vi "Slave_P.vi"() -> ()   [LabVIEW 2017, in "Konfiguracja.lvlib"]
uses:
  Libraries/Konfiguracja/Konfiguracja.lvlib
  Controls/Enum_SM_read_input_write.ctl
  <vilib>/Utility/config.llb/NI_LVConfig.lvlib
panel:
  in  "System Tab":enum32{"Termometry i paliwo"}(tab)
  in  "Etykiety P1-6":T1
  in  "Ratio 6":dbl min=0.0 step=1.0
  in  "Ratio 5":dbl min=0.0 step=1.0
  in  "Ratio 4":dbl min=0.0 step=1.0
  in  "Ratio 3":dbl min=0.0 step=1.0
  in  "Ratio 2":dbl min=0.0 step=1.0
  in  "Ratio 1":dbl min=0.0 step=1.0
  in  "Stan 6":dbl min=0.0 step=1.0
  in  "Stan 5":dbl min=0.0 step=1.0
  in  "Stan 4":dbl min=0.0 step=1.0
  in  "Stan 3":dbl min=0.0 step=1.0
  in  "Stan 2":dbl min=0.0 step=1.0
  in  "Stan 1":dbl min=0.0 step=1.0
  in  "Paliwo 6":bool
  in  "Paliwo 5":bool
  in  "Paliwo 4":bool
  in  "Paliwo 3":bool
  in  "Paliwo 2":bool
  in  "Paliwo 1":bool caption="Termometr 1"
  in  "Moduł aktywny":bool
  in  "Identyfikator slave'a":dbl=2.0 min=2.0 max=127.0 step=1.0
  in  "Copy":bool
  in  "Save":bool
  # "Etykieta"
  # "Stan licznika"
  # "Ratio"
  # "Kopiuje wartośc zadaną z \npola 1 do pozostałych"
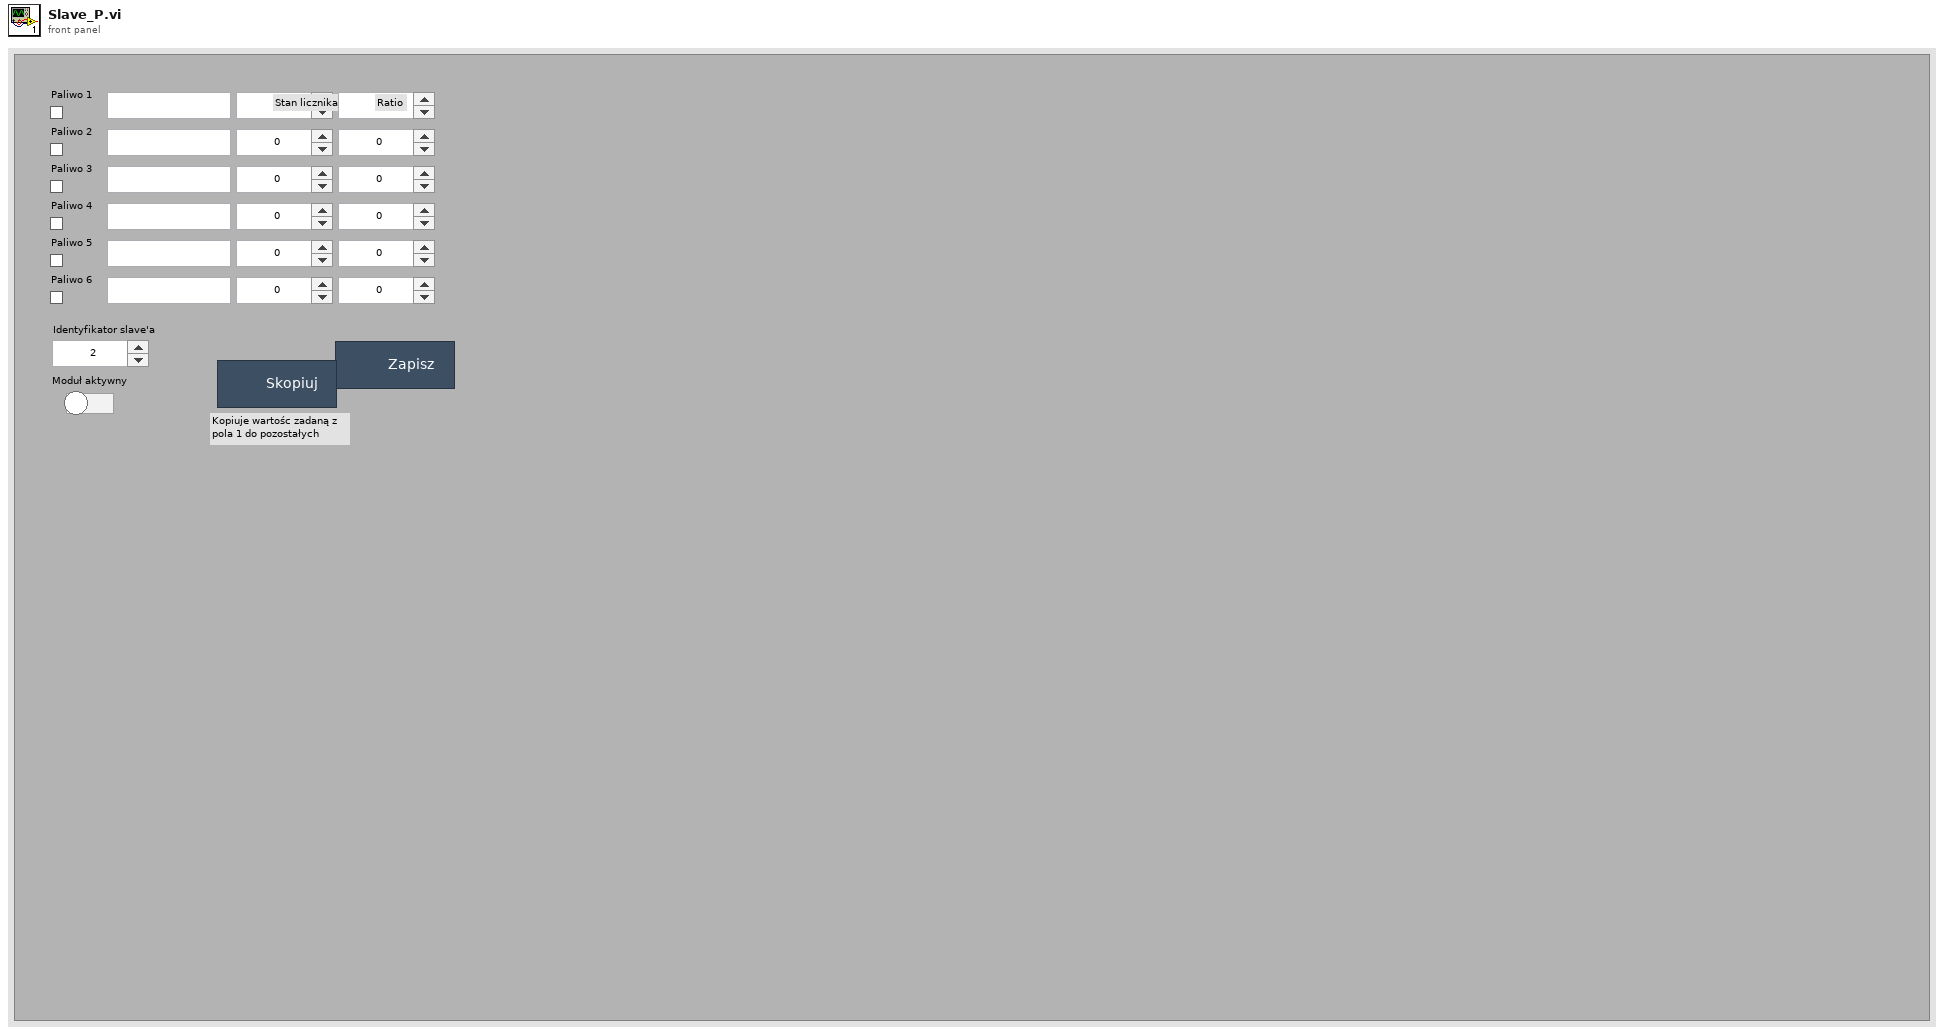
[diagram p1: front panel]
types:
  T1 = cluster{"Paliwo 1":string, "Paliwo 2":string, "Paliwo 3":string, "Paliwo 4":string, "Paliwo 5":string, "Paliwo 6":string}
  T2 = typedef "Konfiguracja.lvlib/Enum_SM_read_input_write.ctl" = enum16{"Load", "Wait for input", "Input", "Copy", "Write", "Exit"}
  T3 = cluster{bool, "P_Sx":cluster{"Stan 1":dbl, "Stan 2":dbl, "Stan 3":dbl, "Stan 4":dbl, "Stan 5":dbl, "Stan 6":dbl}, "P_Rx":cluster{"Ratio 1":dbl, "Ratio 2":dbl, "Ratio 3":dbl, "Ratio 4":dbl, "Ratio 5":dbl, "Ratio 6":dbl}, "Px":cluster{"Paliwo 1":bool, "Paliwo 2":bool, "Paliwo 3":bool, "Paliwo 4":bool, "Paliwo 5":bool, "Paliwo 6":bool}}
  T4 = cluster{"Stan 1":dbl, "Stan 2":dbl, "Stan 3":dbl, "Stan 4":dbl, "Stan 5":dbl, "Stan 6":dbl}
  T5 = cluster{"Ratio 1":dbl, "Ratio 2":dbl, "Ratio 3":dbl, "Ratio 4":dbl, "Ratio 5":dbl, "Ratio 6":dbl}
  T6 = cluster{"Paliwo 1":bool, "Paliwo 2":bool, "Paliwo 3":bool, "Paliwo 4":bool, "Paliwo 5":bool, "Paliwo 6":bool}
  T7 = cluster{cluster{"Paliwo 1":bool, "Paliwo 2":bool, "Paliwo 3":bool, "Paliwo 4":bool, "Paliwo 5":bool, "Paliwo 6":bool}, cluster{"Ratio 1":dbl, "Ratio 2":dbl, "Ratio 3":dbl, "Ratio 4":dbl, "Ratio 5":dbl, "Ratio 6":dbl}, cluster{"Stan 1":dbl, "Stan 2":dbl, "Stan 3":dbl, "Stan 4":dbl, "Stan 5":dbl, "Stan 6":dbl}, "Moduł aktywny":bool, "Etykiety P1-6":cluster{"Paliwo 1":string, "Paliwo 2":string, "Paliwo 3":string, "Paliwo 4":string, "Paliwo 5":string, "Paliwo 6":string}}
  T8 = typedef "NI_LVConfig.lvlib/Config Data RefNum.ctl" = refnum<k1>
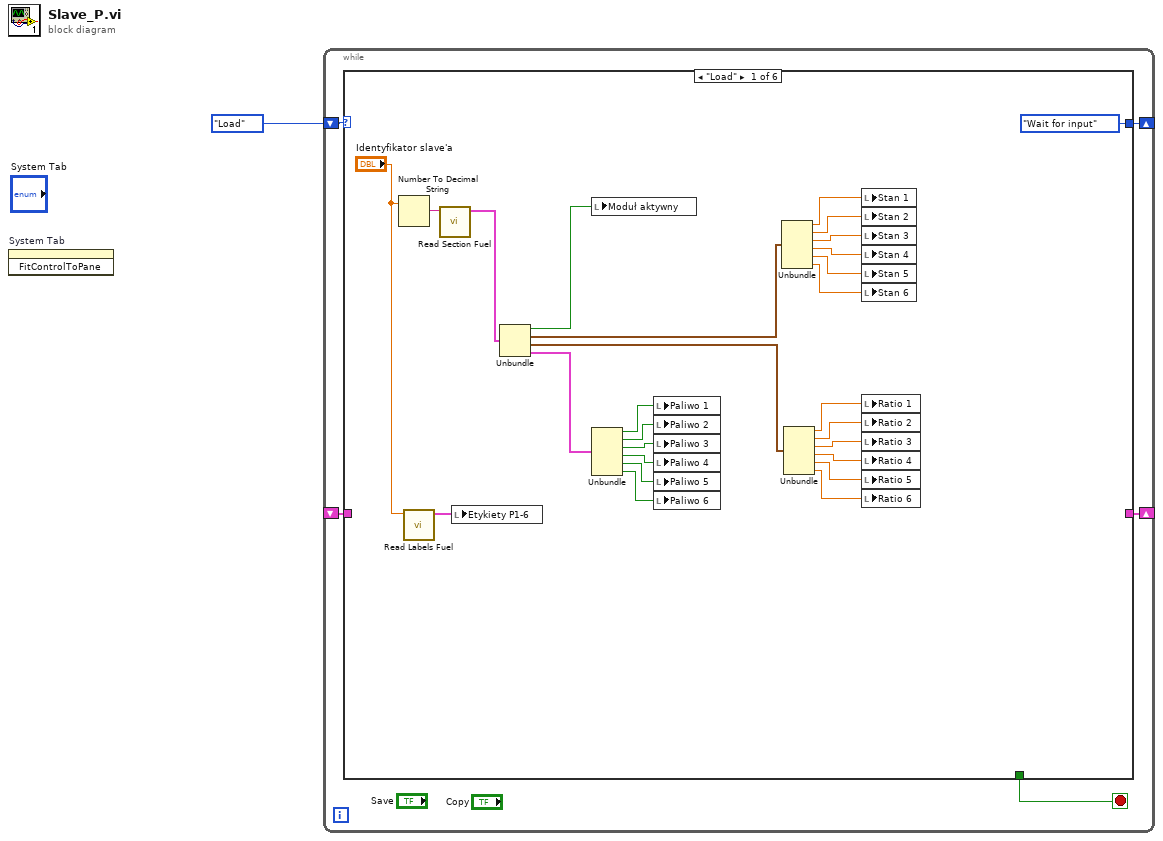
[diagram p0: block diagram]
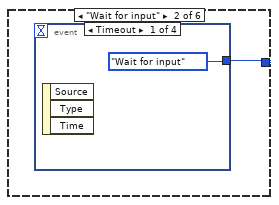
[diagram p2: hidden frame]
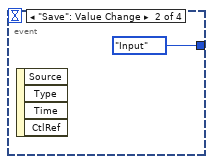
[diagram p3: hidden frame]
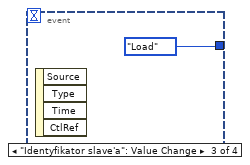
[diagram p4: hidden frame]
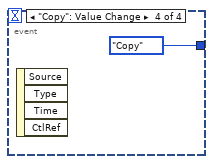
[diagram p5: hidden frame]
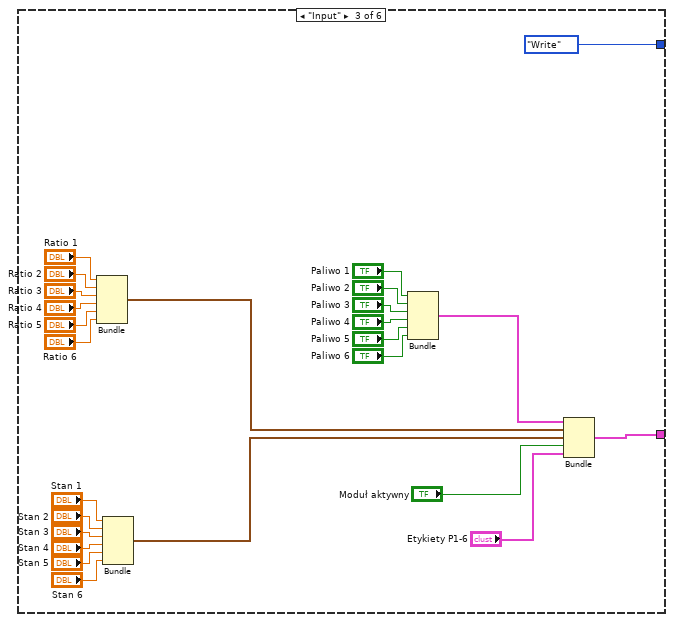
[diagram p6: hidden frame]
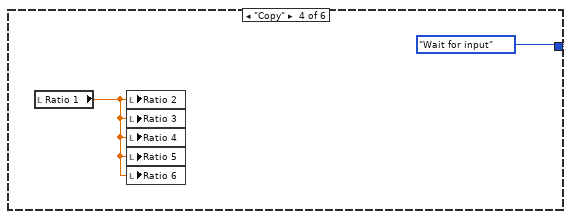
[diagram p7: hidden frame]
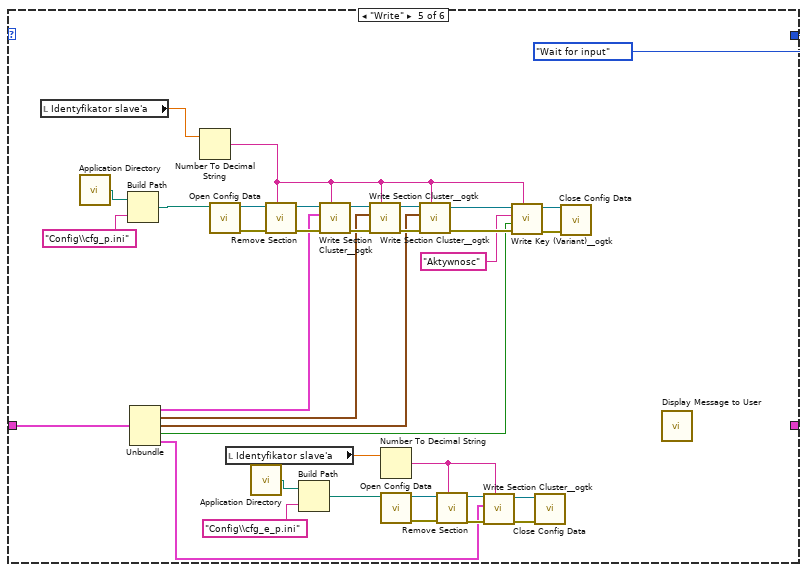
[diagram p8: hidden frame]
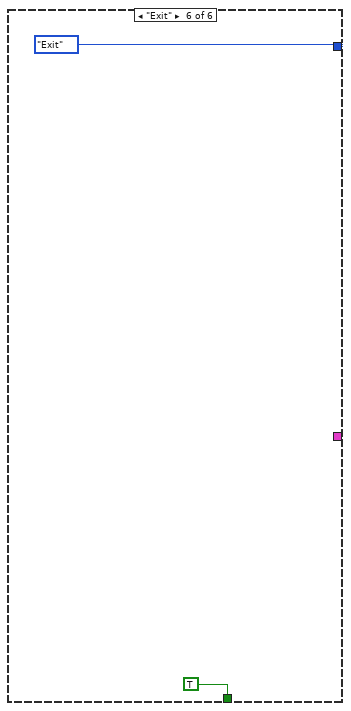
[diagram p9: hidden frame]
diagram:
  n1 = invoke on="System Tab" class="TabCtl (strict)" method="FitControlToPane"() -> ()  [unwired: 3 in, 3 out]
  n2 = while {
    shift-right: [w5] -> _
    shift-left: Enum_SM_read_input_write."Load" -> [w6]
    shift-right: [w4] -> _
    shift-left: _ -> [w3]
    stop <- w2 stop-if-true
    n3 = case shown="\"Load\"" w6 {
      tunnel: [Enum_SM_read_input_write."Wait for input" w34 Enum_SM_read_input_write."Write" Enum_SM_read_input_write."Wait for input" Enum_SM_read_input_write."Wait for input" Enum_SM_read_input_write."Exit"] -> w5
      tunnel: [_ _ w57 _ _ _] -> w4
      tunnel: w3 -> [_ _ _ _ w96 _]
      tunnel: [_ _ _ _ _ TRUE] -> w2
      frame "Load" {
        n4 = Number To Decimal String(number="Identyfikator slave'a") -> (decimal integer string=w20:string)  [unwired: 1 in]
        n5 = call "Read Labels Fuel.vi"("Slave ID"="Identyfikator slave'a") -> ("Etykiety P1-6"=w7:T1)  [unwired: 10 in]
        n6 = call "Read Section Fuel.vi"("section in"=w20) -> ("Data Cluster"=w19:T3)  [unwired: 10 in]
        n7 = local write "Etykiety P1-6"(w7) -> ()
        n8 = Unbundle(w19) -> (w18:bool, "P_Sx"=w17:T4, "P_Rx"=w9:T5, "Px"=w16:T6)
        n9 = local write "Moduł aktywny"(w18) -> ()
        n10 = Unbundle(w16) -> ("Paliwo 1"=w29:bool, "Paliwo 2"=w30:bool, "Paliwo 3"=w32:bool, "Paliwo 4"=w31:bool, "Paliwo 5"=w28:bool, "Paliwo 6"=w27:bool)
        n11 = local write "Paliwo 1"(w29) -> ()
        n12 = local write "Paliwo 2"(w30) -> ()
        n13 = local write "Paliwo 3"(w32) -> ()
        n14 = local write "Paliwo 4"(w31) -> ()
        n15 = local write "Paliwo 5"(w28) -> ()
        n16 = local write "Paliwo 6"(w27) -> ()
        n17 = Unbundle(w17) -> ("Stan 1"=w23:dbl, "Stan 2"=w22:dbl, "Stan 3"=w21:dbl, "Stan 4"=w24:dbl, "Stan 5"=w25:dbl, "Stan 6"=w26:dbl)
        n18 = Unbundle(w9) -> ("Ratio 1"=w12:dbl, "Ratio 2"=w11:dbl, "Ratio 3"=w10:dbl, "Ratio 4"=w13:dbl, "Ratio 5"=w14:dbl, "Ratio 6"=w15:dbl)
        n19 = local write "Stan 1"(w23) -> ()
        n20 = local write "Stan 2"(w22) -> ()
        n21 = local write "Stan 3"(w21) -> ()
        n22 = local write "Stan 4"(w24) -> ()
        n23 = local write "Stan 5"(w25) -> ()
        n24 = local write "Stan 6"(w26) -> ()
        n25 = local write "Ratio 1"(w12) -> ()
        n26 = local write "Ratio 2"(w11) -> ()
        n27 = local write "Ratio 3"(w10) -> ()
        n28 = local write "Ratio 4"(w13) -> ()
        n29 = local write "Ratio 5"(w14) -> ()
        n30 = local write "Ratio 6"(w15) -> ()
      }
      frame "Wait for input" {
        n31 = event shown="[0] Timeout" {
          selector: _ -> [_ _ _ _]
          dyn-events: _ -> [_ _ _ _]
          timeout: _ -> [_ _ _ _]
          tunnel: [Enum_SM_read_input_write."Wait for input" Enum_SM_read_input_write."Input" Enum_SM_read_input_write."Load" Enum_SM_read_input_write."Copy"] -> w34
          event Timeout {
            n32 = event-data() -> ()  [unwired: 1 in, 3 out]
          }
          event "Save": Value Change {
            n33 = event-data() -> ()  [unwired: 1 in, 4 out]
          }
          event "Identyfikator slave'a": Value Change {
            n34 = event-data() -> ()  [unwired: 1 in, 4 out]
          }
          event "Copy": Value Change {
            n35 = event-data() -> ()  [unwired: 1 in, 4 out]
          }
        }
      }
      frame "Input" {
        n36 = Bundle("Ratio 1"="Ratio 1", "Ratio 2"="Ratio 2", "Ratio 3"="Ratio 3", "Ratio 4"="Ratio 4", "Ratio 5"="Ratio 5", "Ratio 6"="Ratio 6") -> (w40:T5)  [unwired: 1 in]
        n37 = Bundle("Stan 1"="Stan 1", "Stan 2"="Stan 2", "Stan 3"="Stan 3", "Stan 4"="Stan 4", "Stan 5"="Stan 5", "Stan 6"="Stan 6") -> (w43:T4)  [unwired: 1 in]
        n38 = Bundle("Paliwo 1"="Paliwo 1", "Paliwo 2"="Paliwo 2", "Paliwo 3"="Paliwo 3", "Paliwo 4"="Paliwo 4", "Paliwo 5"="Paliwo 5", "Paliwo 6"="Paliwo 6") -> (w41:T6)  [unwired: 1 in]
        n39 = Bundle(w41, w40, w43, "Moduł aktywny"="Moduł aktywny", "Etykiety P1-6"="Etykiety P1-6") -> (w57:T7)  [unwired: 1 in]
      }
      frame "Copy" {
        n40 = local read "Ratio 1"() -> (w64:dbl)
        n41 = local write "Ratio 2"(w64) -> ()
        n42 = local write "Ratio 3"(w64) -> ()
        n43 = local write "Ratio 4"(w64) -> ()
        n44 = local write "Ratio 5"(w64) -> ()
        n45 = local write "Ratio 6"(w64) -> ()
      }
      frame "Write" {
        n46 = local read "Identyfikator slave'a"() -> (w84:dbl)
        n47 = call <vilib>:"Application Directory.vi"() -> ("Application Directory"=w99:path)
        n48 = Build Path(base path=w99, name or relative path="Config\\cfg_p.ini") -> (appended path=w97:path)
        n49 = Unbundle(w96) -> (w87:T6, w86:T5, w85:T4, "Moduł aktywny"=w81:bool, "Etykiety P1-6"=w66:T1)
        n50 = Number To Decimal String(number=w84) -> (decimal integer string=w82:string)  [unwired: 1 in]
        n51 = call <vilib>:"Open Config Data.vi"("configuration file path"=w97) -> ("error out"=w88:errorcluster, "refnum"=w91:T8)  [unwired: 8 in, 1 out]
        n52 = local read "Identyfikator slave'a"() -> (w72:dbl)
        n53 = call <vilib>:"Application Directory.vi"() -> ("Application Directory"=w77:path)
        n54 = call <vilib>:"Remove Section.vi"("section"=w82, "error in (no error)"=w88, "refnum"=w91) -> ("error out"=w89:errorcluster, "refnum out"=w90:T8)  [unwired: 6 in, 1 out]
        n55 = Build Path(base path=w77, name or relative path="Config\\cfg_e_p.ini") -> (appended path=w75:path)
        n56 = call <userlib>:"Write Section Cluster__ogtk.vi"("section (optional)"=w82, "error in (no error)"=w89, "Section Formatted Cluster"=w87, "refnum"=w90) -> ("error out"=w93:errorcluster, "dup refnum"=w95:T8)  [unwired: 6 in]
        n57 = call <userlib>:"Write Section Cluster__ogtk.vi"("section (optional)"=w82, "error in (no error)"=w93, "Section Formatted Cluster"=w86, "refnum"=w95) -> ("error out"=w92:errorcluster, "dup refnum"=w94:T8)  [unwired: 6 in]
        n58 = Number To Decimal String(number=w72) -> (decimal integer string=w67:string)  [unwired: 1 in]
        n59 = call <vilib>:"Open Config Data.vi"("configuration file path"=w75) -> ("error out"=w73:errorcluster, "refnum"=w74:T8)  [unwired: 8 in, 1 out]
        n60 = call <userlib>:"Write Section Cluster__ogtk.vi"("section (optional)"=w82, "error in (no error)"=w92, "Section Formatted Cluster"=w85, "refnum"=w94) -> ("error out"=w101:errorcluster, "dup refnum"=w80:T8)  [unwired: 6 in]
        n61 = call <vilib>:"Remove Section.vi"("section"=w67, "error in (no error)"=w73, "refnum"=w74) -> ("error out"=w69:errorcluster, "refnum out"=w68:T8)  [unwired: 6 in, 1 out]
        n62 = call <userlib>:"Write Section Cluster__ogtk.vi"("section (optional)"=w67, "error in (no error)"=w69, "Section Formatted Cluster"=w66, "refnum"=w68) -> ("error out"=w70:errorcluster, "dup refnum"=w71:T8)  [unwired: 6 in]
        n63 = call <userlib>:"Write Key (Variant)__ogtk.vi"("section"=w82, "error in (no error)"=w101, "key-value"=w81, "key (optional)"="Aktywnosc", "refnum"=w80) -> ("error out"=w78:errorcluster, "refnum out"=w79:T8)  [unwired: 5 in]
        n64 = call <vilib>:"Close Config Data.vi"("error in (no error)"=w70, "refnum"=w71) -> ()  [unwired: 8 in, 2 out]
        n65 = call <vilib>:"Close Config Data.vi"("error in (no error)"=w78, "refnum"=w79) -> ()  [unwired: 8 in, 2 out]
        n66 = call "Display Message to User"() -> ()  [unwired: 10 in, 2 out]
      }
      frame "Exit" {
      }
    }
  }
